vi "GetPoint.vi"(8 "error in (no error)":errorcluster, 11 "Point in":refnum<class "Point.lvclass">) -> (0 "error out":errorcluster, 2 "Point":cluster{"x":i16, "y":i16}, 3 "Point out":refnum<class "Point.lvclass">)   [LabVIEW 2021, in "Picture2D.lvlib" / "Point.lvclass"]
uses:
  Point.lvclass
  Point.lvclass/Point.ctl
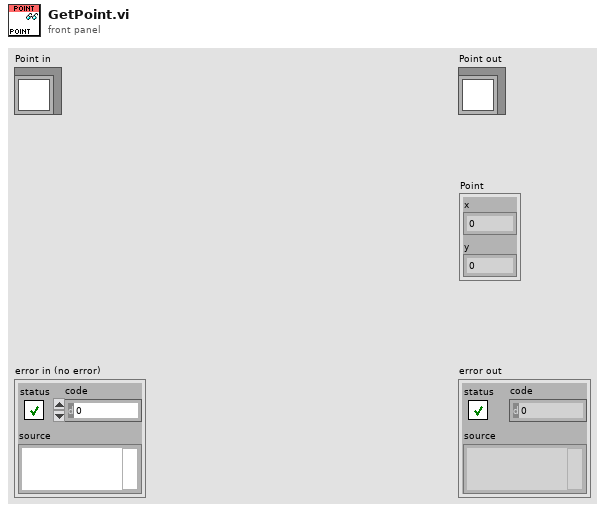
[diagram p1: front panel]
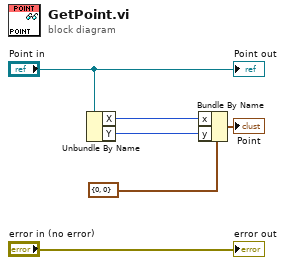
[diagram p0: block diagram]
diagram:
  n1 = Unbundle By Name("Point in") -> ("X"=w2:i16, "Y"=w1:i16)
  n2 = Bundle By Name(cluster=cluster{"x":i16, "y":i16} {"x"=0, "y"=0} ("Point"), "x"=w2, "y"=w1) -> (→"Point":cluster{"x":i16, "y":i16})
  "error out" <- "error in (no error)"
  "Point out" <- "Point in"
